vi "LM model function and gradient (2-Exp, Convolved, Periodic, Fixed Parameters) v3.vi"(3 "output control":T1, 4 "data":variant, 5 "X":dbl[](array[numeric]), 6 "a (with sigma)":dbl[](array[numeric])) -> (0 "error out":errorcluster, 1 "f'(X,a)":dbl[][](array[numeric]), 2 "f(X,a)":dbl[](array[numeric]))   [LabVIEW 2021, in "Fits.lvlib"]
doc: "This template is the starting point for creating a model function to be passed to the Nonlinear Curve Fit.vi."
uses:
  Fits.lvlib
  <vilib>/gmath/NumericalOptimization/LM_output select.ctl
  1-Exp Parameters.ctl
  Fit Control Data v2.ctl
  Graphs/XY Graph/XY Plot Data.ctl
  IRF(X)PSED/Decay Fit Parameters In List.ctl
  Decay Model.ctl
  Graphs/XY Graph/XY Graph Add-Ons.lvlib
  e69e6f48-ad21-4fab-bc0f-ff4b1b8ea852.vi
  <vilib>/gmath/NI_Gmath.lvlib
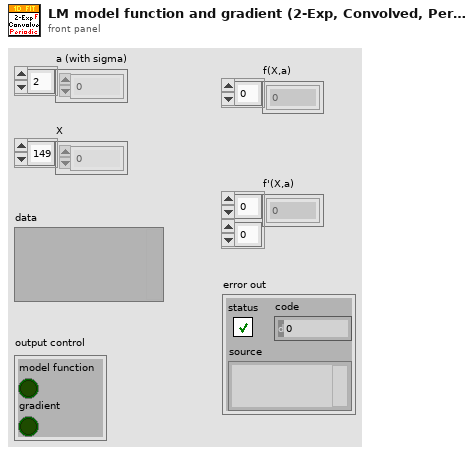
[diagram p1: front panel]
types:
  T1 = typedef "NI_Gmath.lvlib/LM_output select.ctl" = cluster{"model function":bool, "gradient":bool}
  T2 = typedef "Fits.lvlib/1-Exp Parameters.ctl" = cluster{"t_0":dbl, "B":dbl, "A":dbl, "tau":dbl, "T":dbl, "sigma":dbl}
  T3 = typedef "Fits.lvlib/Fit Control Data v2.ctl" = cluster{"IRF":T4, "Laser Period":dbl, "SYNC Period":dbl, "Fixed Parameter Names":T5[], "Fixed Parameter Values":dbl[], "Fitted Parameter Names":T5[], "Fit Model":T6}
  T4 = typedef "XY Graph Add-Ons.lvlib/XY Plot Data.ctl" = cluster{"X Array":dbl[], "Y Array":dbl[]}
  T5 = typedef "Fits.lvlib/Decay Fit Parameters In List.ctl" = enum16{"Offset", "Baseline", "A_1", "tau_1", "A_2", "tau_2"}
  T6 = typedef "Fits.lvlib/Decay Model.ctl" = enum16{"1-Exponential", "2-Exponentials"}
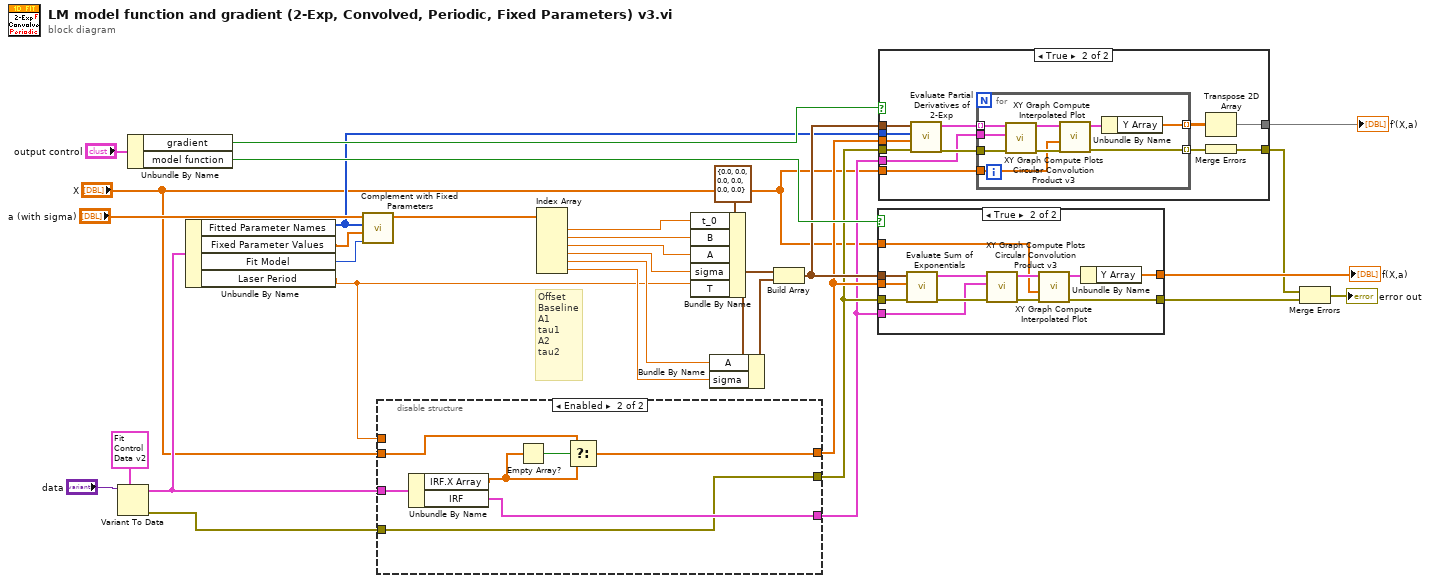
[diagram p0: block diagram]
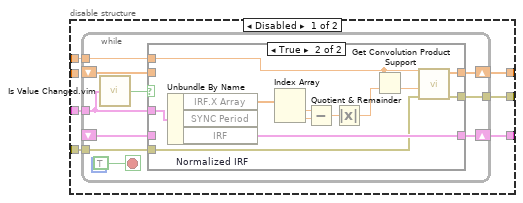
[diagram p2: hidden frame]
diagram:
  # "Offset\nBaseline\nA1\ntau1\nA2\ntau2"
  n1 = Variant To Data(type=T3 {"IRF"={"X Array"=[], "Y Array"=[]}, "Laser Period"=0.0, "SYNC Period"=0.0, "Fixed Parameter Names"=[], "Fixed Parameter Values"=[], "Fitted Parameter Names"=[], "Fit Model"=enum."1-Exponential"} ("Fit Control Data"), Variant="data") -> (data=w16:T3, error out=w3:errorcluster)  [unwired: 1 in]
  n2 = Unbundle By Name("output control") -> ("gradient"=w12:bool, "model function"=w13:bool)
  n3 = Unbundle By Name(w16) -> ("Fitted Parameter Names"=w10:T5[], "Fixed Parameter Values"=w19:dbl[], "Fit Model"=w20:T6, "Laser Period"=w2:dbl)
  n4 = call "Complement with Fixed Parameters.vi"("Fit Model"=w20, "Fixed Parameter Values"=w19, "Fitted Parameter Names"=w10, "a in"="a (with sigma)") -> ("a out"=w17:dbl[])  [unwired: 7 in]
  n5 = disable-structure shown="Enabled" {
    disable-tunnel: w16 -> [w38 w70]
    disable-tunnel: [w37 w65] -> w9
    disable-tunnel: [w36 w68] -> w8
    disable-tunnel: [w35 w69] -> w7
    disable-tunnel: w3 -> [w34 w68]
    disable-tunnel: w2 -> [w33 _]
    disable-tunnel: "X" -> [_ w64]
    frame Disabled {
      n6 = while {
        tunnel: w38 -> [w44]
        tunnel: w34 -> [w47]
        tunnel: [w46] -> w36
        shift-right: [w45] -> w37
        shift-left: _ -> [w41]
        shift-right: [w48] -> w35
        shift-left: _ -> [w40]
        tunnel: w33 -> [w39]
        stop <- TRUE stop-if-true
        n7 = call "Is Value Changed.vim"("value"=w44) -> ("changed or first call?"=w42:bool)
        n8 = case shown="True" w42 {
          tunnel: [w49 w63] -> w48
          tunnel: w47 -> [w50 w56]
          tunnel: [w50 w55] -> w46
          tunnel: [w51 w54] -> w45
          tunnel: w44 -> [_ w53]
          tunnel: w41 -> [w51 _]
          tunnel: w40 -> [w49 _]
          tunnel: w39 -> [_ w52]
          frame False {
          }
          frame True {
            n9 = Unbundle By Name "Normalized IRF"(w53) -> ("IRF.X Array"=w62:dbl[], "IRF"=w63:T4)  [unwired: 1 out]
            n10 = Index Array(array=w62) -> (element #1=w61:dbl, element #2=w60:dbl)  [unwired: 2 in]
            n11 = Subtract(x=w61, y=w60) -> (x-y=w59:dbl)
            n12 = Absolute Value(x=w59) -> (abs(x)=w58:dbl)
            n13 = Quotient & Remainder(x=w52, y=w58) -> (floor(x/y)=w57:dbl)  [unwired: 1 out]
            n14 = call "Get Convolution Product Support.vi"("Error In"=w56, "# Values"=w57, "IRF Period"=w52) -> ("Error Out"=w55:errorcluster, "Ramp"=w54:dbl[])  [unwired: 6 in, 1 out]
          }
        }
      }
    }
    frame Enabled {
      n15 = Unbundle By Name(w70) -> ("IRF.X Array"=w66:dbl[], "IRF"=w69:T4)
      n16 = Empty Array?(array=w66) -> (empty?=w67:bool)
      n17 = Select(t=w64, s=w67, f=w66) -> (s? t:f=w65:dbl[])
    }
  }
  n18 = Index Array(array=w17) -> (element #1=w30:dbl, element #2=w4:dbl, element #3=w28:dbl, element #4=w27:dbl, element #5=w25:dbl, element #6=w24:dbl)  [unwired: 6 in]
  n19 = Bundle By Name(cluster=T2 {"t_0"=0.0, "B"=0.0, "A"=0.0, "tau"=0.0, "T"=0.0, "sigma"=0.0} ("1-Exp Parameters"), "t_0"=w30, "B"=w4, "A"=w28, "sigma"=w27, "T"=w2) -> (w22:T2)
  n20 = Bundle By Name(cluster=w22, "A"=w25, "sigma"=w24) -> (w23:T2)
  n21 = Build Array(w22, w23) -> (w11:T2[])
  n22 = case shown="True" w13 {
    tunnel: [_ w76] -> w29
    tunnel: w11 -> [_ w79]
    tunnel: w9 -> [_ w78]
    tunnel: w8 -> [w71 w77]
    tunnel: [w71 w75] -> w21
    tunnel: w7 -> [_ w73]
    tunnel: "X" -> [_ w72]
    frame False {
    }
    frame True {
      n23 = call "Evaluate Sum of Exponentials.vi"("error in (no error)"=w77, "Ramp"=w78, "Exp Parameters Array"=w79) -> ("error out"=w80:errorcluster, "Plot"=w74:T4)  [unwired: 7 in]
      n24 = call "XY Graph Compute Plots Circular Convolution Product v3.vi"("Error In"=w80, "Plot 2 (kernel)"=w73, "Plot 1 (function)"=w74) -> ("Error Out"=w83:errorcluster, "Convolution Product"=w81:T4)  [unwired: 6 in, 1 out]
      n25 = call "XY Graph Compute Interpolated Plot.vi"("Error In"=w83, "Ramp"=w72, "Plot"=w81) -> ("Error Out"=w75:errorcluster, "Interpolated Plot"=w82:T4)  [unwired: 7 in]
      n26 = Unbundle By Name(w82) -> ("Y Array"=w76:dbl[])
    }
  }
  "f(X,a)" <- w29
  n27 = case shown="True" w12 {
    tunnel: w11 -> [_ w96]
    tunnel: w10 -> [_ w95]
    tunnel: w8 -> [w84 w94]
    tunnel: w9 -> [_ w92]
    tunnel: [_ w89] -> w6
    tunnel: "X" -> [_ w88]
    tunnel: w7 -> [_ w87]
    tunnel: [w84 w85] -> w5
    frame False {
    }
    frame True {
      n28 = call "Evaluate Partial Derivatives of 2-Exp.vi"("error in (no error)"=w94, "Ramp"=w92, "Fitted Parameter Names"=w95, "1-Exp Parameters Array"=w96) -> ("error out"=w91:errorcluster, "Partial Derivatives Plot Array"=w93:T4[])  [unwired: 6 in]
      n29 = for {
        tunnel: w93 -> [w105] mode=indexing
        tunnel: w87 -> [w104]
        tunnel: w91 -> [w103]
        tunnel: w88 -> [w100]
        tunnel: [w98] -> w90 mode=indexing
        tunnel: [w97] -> w86 mode=indexing
        n30 = call "XY Graph Compute Plots Circular Convolution Product v3.vi"("Error In"=w103, "Plot 2 (kernel)"=w104, "Plot 1 (function)"=w105) -> ("Error Out"=w102:errorcluster, "Convolution Product"=w101:T4)  [unwired: 6 in, 1 out]
        n31 = call "XY Graph Compute Interpolated Plot.vi"("Error In"=w102, "Ramp"=w100, "Plot"=w101) -> ("Error Out"=w97:errorcluster, "Interpolated Plot"=w99:T4)  [unwired: 7 in]
        n32 = Unbundle By Name(w99) -> ("Y Array"=w98:dbl[])
      }
      n33 = Transpose 2D Array(2D array=w90) -> (transposed array=w89:dbl[][])
      n34 = Merge Errors(w86) -> (w85:errorcluster)
    }
  }
  "f'(X,a)" <- w6
  n35 = Merge Errors(w5, w21) -> (→"error out":errorcluster)
